vi "Bounds Fixed.vi"(8 "+/-":dbl, 11 "Nominal":dbl) -> (0 "Min":dbl, 3 "Max":dbl)   [LabVIEW 2019]
doc: "This VI simply calcualtes the toleance limits given the \"Nominal\" and \"+/-\" values."
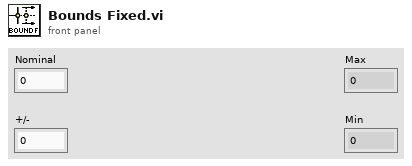
[diagram p1: front panel]
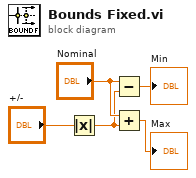
[diagram p0: block diagram]
diagram:
  n1 = Absolute Value(x="+/-") -> (abs(x)=w3:dbl)
  n2 = Subtract(x="Nominal", y=w3) -> (x-y=→"Min":dbl)
  n3 = Add(x="Nominal", y=w3) -> (x+y=→"Max":dbl)
